vi "Terminate.vi"(8 "error in (no error)":errorcluster, 11 "ATM Controller in":refnum<class "ATM Controller.lvclass">) -> (0 "error out":errorcluster, 3 "ATM Controller out":refnum<class "ATM Controller.lvclass">)   [LabVIEW 2020, in "ATM Controller.lvclass"]
uses:
  ATM Controller.lvclass
  ATM Controller.lvclass/ATM Controller.ctl
  State.ctl
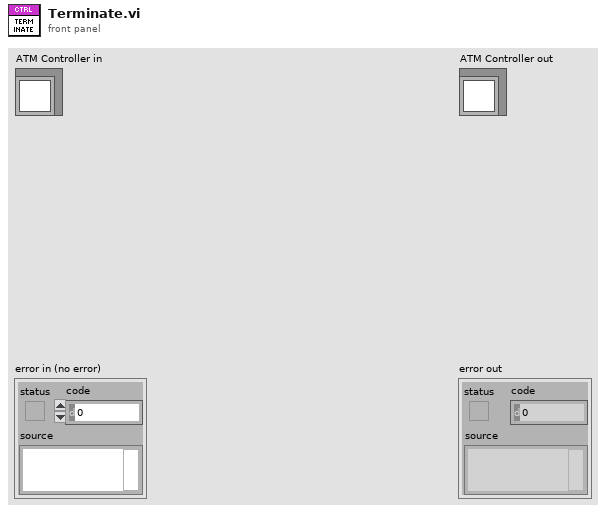
[diagram p1: front panel]
types:
  T1 = typedef "ATM Controller.lvclass/State.ctl" = enum16{"Start", "Card Inserted", "Verification Failed", "Verification Succeeded", "Depositing", "Depositing Completed", "Withdrawing", "Withdraw Completed", "Withdraw Failed", "Balance Inquiry", "Terminate"}
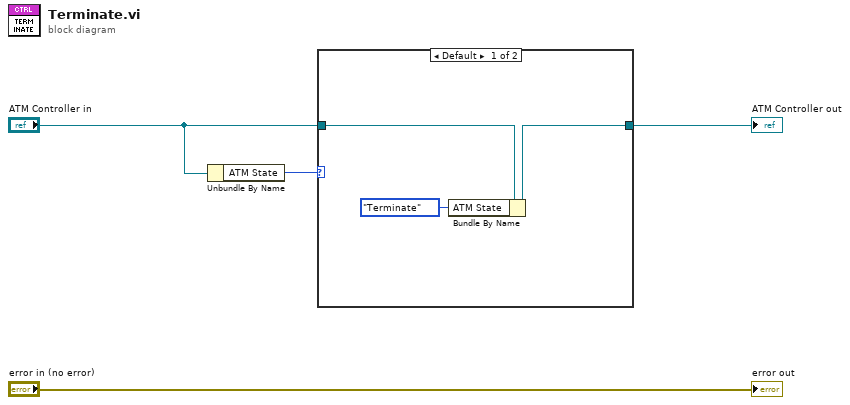
[diagram p0: block diagram]
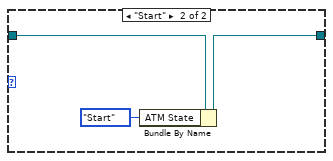
[diagram p2: hidden frame]
diagram:
  n1 = Unbundle By Name("ATM Controller in") -> ("ATM State"=w1:T1)
  n2 = case shown="Default" w1 {
    tunnel: "ATM Controller in" -> [w7 w10]
    tunnel: [w6 w9] -> w2
    frame Default {
      n3 = Bundle By Name(cluster=w7, "ATM State"=State."Terminate") -> (w6:refnum<class "ATM Controller.lvclass">)
    }
    frame "Start" {
      n4 = Bundle By Name(cluster=w10, "ATM State"=State."Start") -> (w9:refnum<class "ATM Controller.lvclass">)
    }
  }
  "ATM Controller out" <- w2
  "error out" <- "error in (no error)"
